vi "API Testing.vi"() -> ()   [LabVIEW 2023, in "Thermotron 8800.lvlib"]
uses:
  Thermotron 8800.lvlib
panel:
  in  "On/Off":bool
  in  "stop":bool
  out "Temperature Feedback":string
  out "error out":errorcluster
  in  "Temperature Upper Limit":dbl=100.0 min=-200.0 max=300.0 step=1.0 format="%.1f"
  in  "Temperature Lower Limit":dbl min=-200.0 max=300.0 step=1.0 format="%.1f"
  in  "error in (no error)":errorcluster
  in  "Temperature Setpoint":dbl=25.0 min=-200.0 max=300.0 step=1.0 format="%.1f"
  in  "VISA resource name":refnum<visa-resource-name>="TCPIP::127.0.0.1::8888::SOCKET"
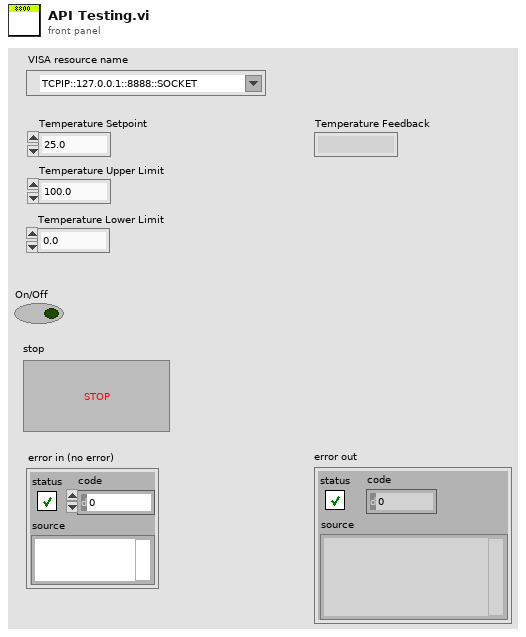
[diagram p1: front panel]
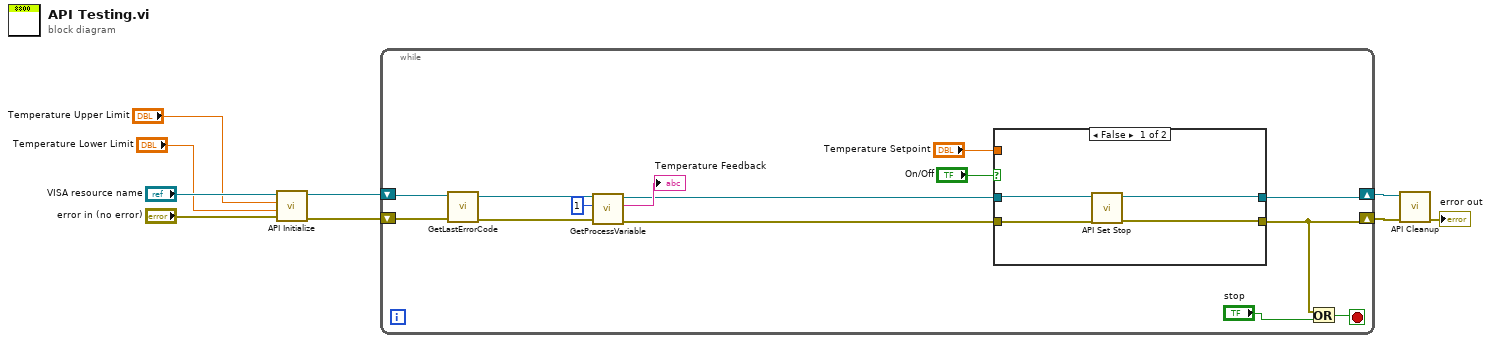
[diagram p0: block diagram]
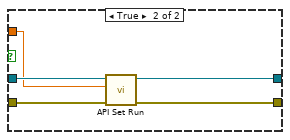
[diagram p2: hidden frame]
diagram:
  n1 = call "API Initialize.vi"("error in (no error)"="error in (no error)", "Temperature Lower Limit"="Temperature Lower Limit", "Temperature Upper Limit"="Temperature Upper Limit", "VISA resource name"="VISA resource name") -> ("error out"=w4:errorcluster, "VISA resource name out"=w3:refnum<visa-resource-name>)  [unwired: 6 in]
  n2 = while {
    shift-right: [w10] -> w2
    shift-left: w4 -> [w17]
    shift-right: [w11] -> w1
    shift-left: w3 -> [w16]
    stop <- w21 stop-if-true
    n3 = call "GetLastErrorCode.vi"("error in"=w17, "VISA resource name"=w16) -> ("error out"=w14:errorcluster, "VISA resource name out"=w15:refnum<visa-resource-name>)  [unwired: 6 in, 2 out]
    n4 = call "GetProcessVariable.vi"("error in"=w14, "Channel (1-140)"=u16 1, "VISA resource name"=w15) -> ("error out"=w13:errorcluster, "Process Variable"=→"Temperature Feedback":string, "VISA resource name out"=w12:refnum<visa-resource-name>)  [unwired: 5 in, 1 out]
    n5 = case shown="False" "On/Off" {
      tunnel: "Temperature Setpoint" -> [_ w30]
      tunnel: w13 -> [w26 w32]
      tunnel: w12 -> [w27 w31]
      tunnel: [w25 w29] -> w11
      tunnel: [w24 w28] -> w10
      frame False {
        n6 = call "API Set Stop.vi"("error in"=w26, "VISA resource name"=w27) -> ("error out"=w24:errorcluster, "VISA resource name out"=w25:refnum<visa-resource-name>)  [unwired: 8 in]
      }
      frame True {
        n7 = call "API Set Run.vi"("error in"=w32, "Air Temperature Setpoint"=w30, "VISA resource name"=w31) -> ("error out"=w28:errorcluster, "VISA resource name out"=w29:refnum<visa-resource-name>)  [unwired: 7 in]
      }
    }
    n8 = Or(x=w10, y="stop") -> (x .or. y?=w21:bool)
  }
  n9 = call "API Cleanup.vi"("error in"=w2, "VISA resource name"=w1) -> ("error out"=→"error out":errorcluster)  [unwired: 9 in]
